vi "Outputs FX Read.vi"(8 "Error":errorcluster, 9 "Read Closed Loop":bool, 11 "Ref":T5) -> (0 "Error Out":errorcluster, 2 "Sensor Values Out":T1, 3 "DevRef Out":T5)   [LabVIEW 2020, in "Grabber_ACT.lvlib"]
uses:
  Grabber_ACT.lvlib
  <vilib>/Rock Robotics/WPI/MotorControl/WPI_MotorControlDeviceRef.ctl
  <vilib>/Rock Robotics/WPI/MotorControl/WPI_MotorControlType.ctl
  <vilib>/Rock Robotics/SystemInterfaces/DIO/FPGA_DIOPWMChannel.ctl
  <vilib>/Rock Robotics/WPI/PWM/WPI_PWMDeadband.ctl
  <vilib>/Rock Robotics/SystemInterfaces/DIO/FPGA_DIOChannel.ctl
  Shared Code/TypeDefs/Cluster_Grabber HW Outputs.ctl
  Shared Code/TypeDefs/Cluster_FX Sensor Values.ctl
  Shared Code/TypeDefs/Cluster_FX CloseLoop Values.ctl
  Shared Code/TypeDefs/Cluster_FX Current Values.ctl
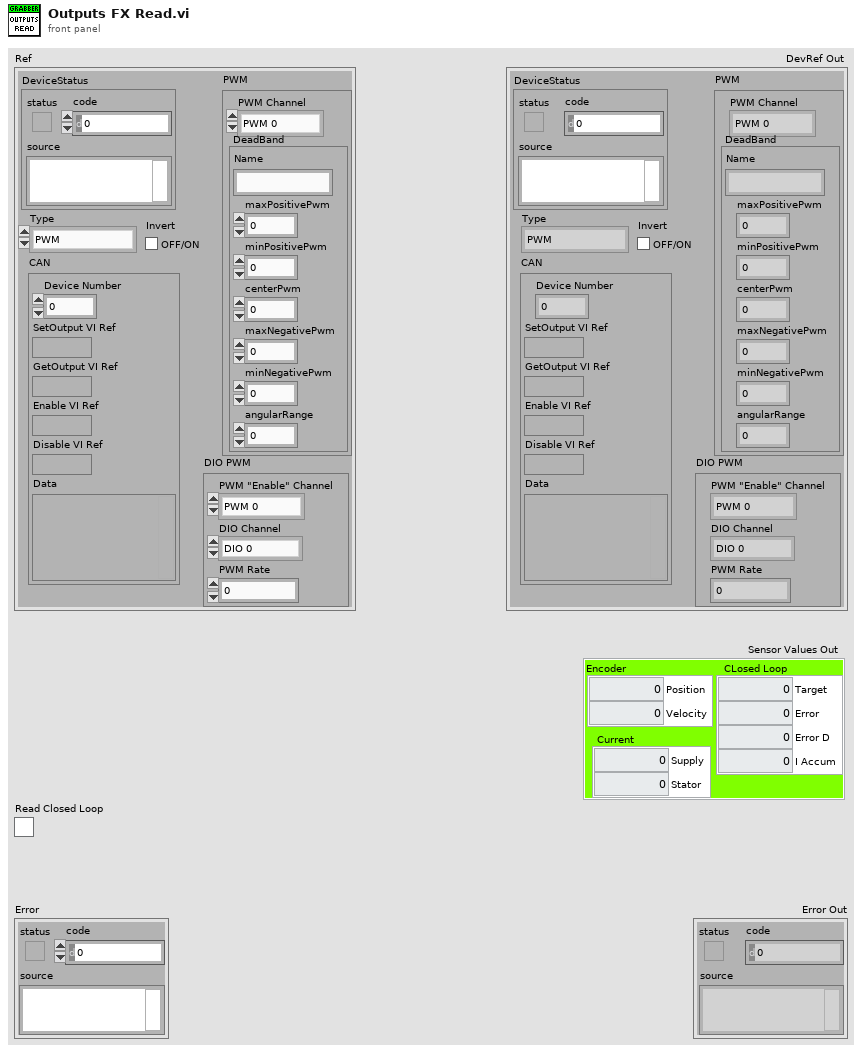
[diagram p1: front panel]
types:
  T1 = typedef "Cluster_Grabber HW Outputs.ctl" = cluster{"Encoder":T2, "CLosed Loop":T3, "Current":T4}
  T2 = typedef "Cluster_FX Sensor Values.ctl" = cluster{"Position":i32, "Velocity":i32}
  T3 = typedef "Cluster_FX CloseLoop Values.ctl" = cluster{"Target":dbl, "Error":i32, "Error D":dbl, "I Accum":dbl}
  T4 = typedef "Cluster_FX Current Values.ctl" = cluster{"Supply":dbl, "Stator":dbl}
  T5 = typedef "WPI_MotorControlDeviceRef.ctl" = cluster{"DeviceStatus":errorcluster, "Type":T6, "PWM":cluster{"PWM Channel":T7, "DeadBand":T8}, "CAN":cluster{"Device Number":u8, "SetOutput VI Ref":variant, "GetOutput VI Ref":variant, "Enable VI Ref":variant, "Disable VI Ref":variant, "Data":variant}, "Invert":bool, "DIO PWM":cluster{"PWM \"Enable\" Channel":T7, "DIOChannel":T9, "PWM Rate":dbl}}
  T6 = typedef "WPI_MotorControlType.ctl" = enum16{"PWM", "CAN", "DIO PWM"}
  T7 = typedef "FPGA_DIOPWMChannel.ctl" = enum8{"PWM 0", "PWM 1", "PWM 2", "PWM 3", "PWM 4", "PWM 5", "PWM 6", "PWM 7", "PWM 8", "PWM 9", "PWM MXP 0", "PWM MXP 1", "PWM MXP 2", "PWM MXP 3", "PWM MXP 4", "PWM MXP 5", "PWM MXP 6", "PWM MXP 7", "PWM MXP 8", "PWM MXP 9", "Invalid"}
  T8 = typedef "WPI_PWMDeadband.ctl" = cluster{"Name":string, "maxPositivePwm":i32, "minPositivePwm":i32, "centerPwm":i32, "maxNegativePwm":i32, "minNegativePwm":i32, "angularRange":u16}
  T9 = typedef "FPGA_DIOChannel.ctl" = enum8{"DIO 0", "DIO 1", "DIO 2", "DIO 3", "DIO 4", "DIO 5", "DIO 6", "DIO 7", "DIO 8", "DIO 9", "DIO MXP 0", "DIO MXP 1", "DIO MXP 2", "DIO MXP 3", "DIO MXP 4", "DIO MXP 5", "DIO MXP 6", "DIO MXP 7", "DIO MXP 8", "DIO MXP 9", "DIO MXP 10", "DIO MXP 11", "DIO MXP 12", "DIO MXP 13", "DIO MXP 14", "DIO MXP 15", "SPI Port CS1", "SPI Port CS2", "SPI Port CS3", "SPI Port MISO", "SPI Port MOSI", "Invalid"}
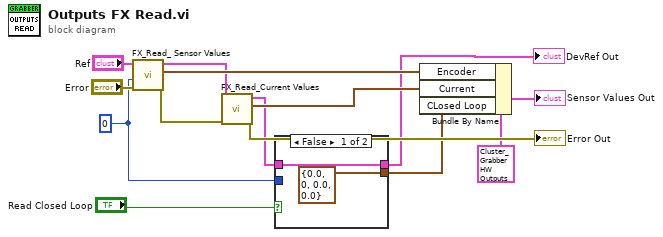
[diagram p0: block diagram]
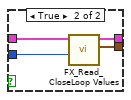
[diagram p2: hidden frame]
diagram:
  w4 = u32 0 ("PidLoopIdx")
  n1 = call "FX_Read_ Sensor Values.vi"("Error"="Error", "PidLoopIdx"=w4, "PhoenixMotorControlDevRef"="Ref") -> ("Error Out"=w1:errorcluster, "Encoder Values Out"=w9:T2, "PhoenixMotorControlDevRef Out"=w2:T5)  [unwired: 6 in]
  n2 = call "FX_Read_Current Values.vi"("error in"=w1, "PhoenixMotorControlDevRef in"=w2) -> ("error out"=→"Error Out":errorcluster, "Current Values"=w8:T4, "PhoenixMotorControlDevRef out"=w7:T5)  [unwired: 7 in]
  n3 = case shown="False" "Read Closed Loop" {
    tunnel: w7 -> [w16 w20]
    tunnel: [w16 w19] -> w6
    tunnel: [T3 {"Target"=0.0, "Error"=0, "Error D"=0.0, "I Accum"=0.0} ("CLosed Loop Out") w18] -> w5
    tunnel: w4 -> [_ w17]
    frame False {
    }
    frame True {
      n4 = call "FX_Read_CloseLoop Values.vi"("Slot"=w17, "PhoenixMotorControlDevRef"=w20) -> ("CLosed Loop Out"=w18:T3, "PhoenixMotorControlDevRef Out"=w19:T5)  [unwired: 7 in, 1 out]
    }
  }
  "DevRef Out" <- w6
  n5 = Bundle By Name(cluster=T1 {"Encoder"={"Position"=0, "Velocity"=0}, "CLosed Loop"={"Target"=0.0, "Error"=0, "Error D"=0.0, "I Accum"=0.0}, "Current"={"Supply"=0.0, "Stator"=0.0}} ("Sensor Values Out"), "Encoder"=w9, "Current"=w8, "CLosed Loop"=w5) -> (→"Sensor Values Out":T1)
